vi "ep_Generate Fundamental Components.vi"(0 "nominal sampling rate (Hz)":u16=9600, 5 "nominal frequency value":dbl=50.0) -> (4 "cos - j*sin":cdb[](array[numeric]))   [LabVIEW 2011, in "NI_EP_Power Quality.lvlib"]
uses:
  <vilib>/addons/Electrical Power/PQ/NI_EP_Power Quality.lvlib
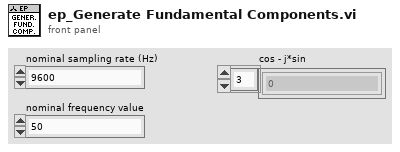
[diagram p1: front panel]
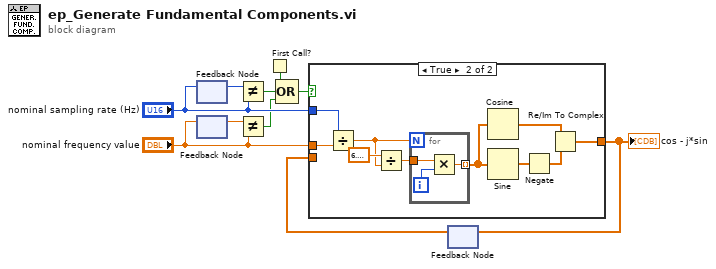
[diagram p0: block diagram]
diagram:
  n1 = feedback-in #1("nominal sampling rate (Hz)") -> ()
  n2 = feedback #1() -> (w9:u16)  [unwired: 1 in]
  n3 = feedback-in #2("nominal frequency value") -> ()
  n4 = feedback #2() -> (w4:dbl)  [unwired: 1 in]
  n5 = Not Equal?(x=w9, y="nominal sampling rate (Hz)") -> (x != y?=w6:bool)
  n6 = Not Equal?(x=w4, y="nominal frequency value") -> (x != y?=w2:bool)
  n7 = First Call?() -> (First Call?: T/F=w7:bool)
  n8 = Compound Arithmetic op=OR(w7, w6, w2) -> (w5:bool)
  n9 = feedback #3() -> (w1:cdb[])  [unwired: 1 in]
  n10 = case shown="True" w5 {
    tunnel: [w11 w13] -> w10
    tunnel: w1 -> [w11 _]
    tunnel: "nominal frequency value" -> [_ w12]
    tunnel: "nominal sampling rate (Hz)" -> [_ w17]
    frame False {
    }
    frame True {
      n11 = Divide(x=w17, y=w12) -> (x/y=w16:dbl)
      n12 = Divide(x=6.283185307179586, y=w16) -> (x/y=w21:dbl)
      n13 = for {
        N: w16 -> [_]
        tunnel: w21 -> [w24]
        tunnel: [w22] -> w19 mode=indexing
        i -> [w23]
        n14 = Multiply(x=w24, y=w23) -> (x*y=w22:dbl)
      }
      n15 = Cosine(x=w19) -> (cos(x)=w14:dbl[])
      n16 = Sine(x=w19) -> (sin(x)=w20:dbl[])
      n17 = Negate(x=w20) -> (-x=w15:dbl[])
      n18 = Re/Im To Complex(1:w15, 2:w14) -> (0:w13:cdb[])
    }
  }
  "cos - j*sin" <- w10
  n19 = feedback-in #3(w10) -> ()
